vi "Create Queue.vi"(9 "Queue":refnum<class "Queue.lvclass">, 10 "Self Queue Alias":string, 11 "Create Queue in":refnum<class "Create Queue.lvclass">) -> (3 "Create Queue out":refnum<class "Create Queue.lvclass">)   [LabVIEW 2021, in "Create Queue Msg Strategy.lvlib" / "Create Queue.lvclass"]
uses:
  Create Queue.lvclass
  jettl/Queue/Queue.lvclass
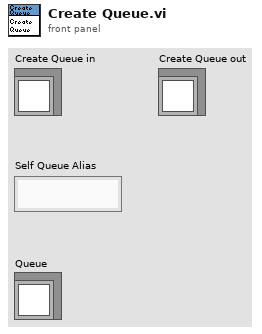
[diagram p1: front panel]
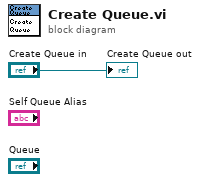
[diagram p0: block diagram]
diagram:
  "Create Queue out" <- "Create Queue in"
